vi "Adjacent Locations.vi"(2 "Current Location":cdb) -> (5 "4 Adjacent Locations":T2, 6 "8 Adjacent Locations":T1)   [LabVIEW 2020]
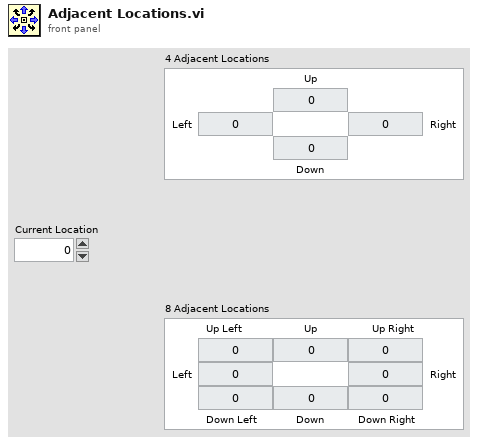
[diagram p1: front panel]
types:
  T1 = cluster{"Up":cdb, "Down":cdb, "Right":cdb, "Left":cdb, "Up Right":cdb, "Up Left":cdb, "Down Right":cdb, "Down Left":cdb}
  T2 = cluster{"Up":cdb, "Down":cdb, "Right":cdb, "Left":cdb}
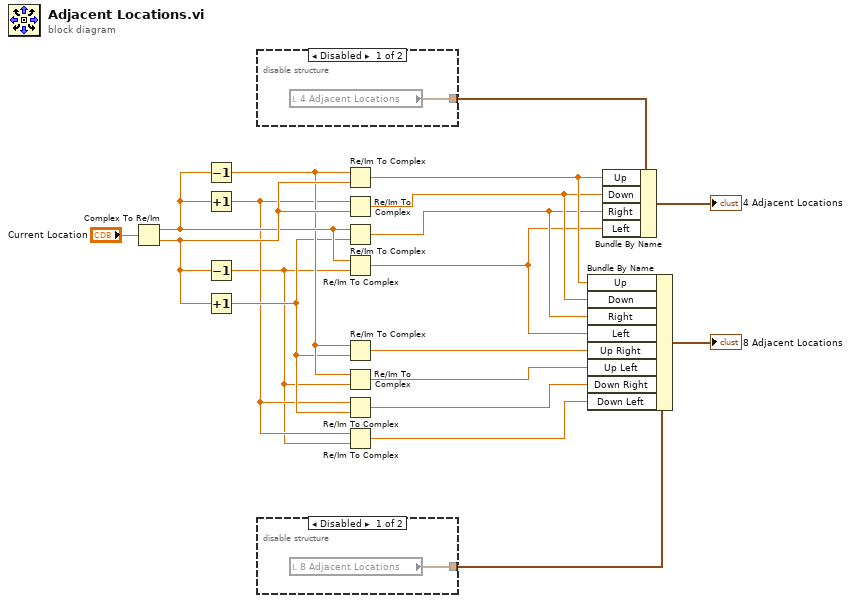
[diagram p0: block diagram]
diagram:
  n1 = Complex To Re/Im(x + iy="Current Location") -> (x=w18:dbl, y=w19:dbl)
  n2 = Decrement(x=w18) -> (x-1=w7:dbl)
  n3 = Increment(x=w18) -> (x+1=w5:dbl)
  n4 = Decrement(x=w19) -> (x-1=w4:dbl)
  n5 = Increment(x=w19) -> (x+1=w6:dbl)
  n6 = disable-structure shown="Disabled" {
    disable-tunnel: [w20 _] -> w15
    frame Disabled {
      n7 = local read "4 Adjacent Locations"() -> (w20:T2)
    }
    frame Enabled {
    }
  }
  n8 = disable-structure shown="Disabled" {
    disable-tunnel: [w21 _] -> w14
    frame Disabled {
      n9 = local read "8 Adjacent Locations"() -> (w21:T1)
    }
    frame Enabled {
    }
  }
  n10 = Re/Im To Complex(1:w19, 2:w7) -> (0:w12:cdb)
  n11 = Re/Im To Complex(1:w19, 2:w5) -> (0:w11:cdb)
  n12 = Re/Im To Complex(1:w6, 2:w18) -> (0:w10:cdb)
  n13 = Re/Im To Complex(1:w4, 2:w18) -> (0:w9:cdb)
  n14 = Re/Im To Complex(1:w6, 2:w7) -> (0:w8:cdb)
  n15 = Re/Im To Complex(1:w4, 2:w7) -> (0:w3:cdb)
  n16 = Re/Im To Complex(1:w6, 2:w5) -> (0:w2:cdb)
  n17 = Re/Im To Complex(1:w4, 2:w5) -> (0:w1:cdb)
  n18 = Bundle By Name(cluster=w14, "Up"=w12, "Down"=w11, "Right"=w10, "Left"=w9, "Up Right"=w8, "Up Left"=w3, "Down Right"=w2, "Down Left"=w1) -> (→"8 Adjacent Locations":T1)
  n19 = Bundle By Name(cluster=w15, "Up"=w12, "Down"=w11, "Right"=w10, "Left"=w9) -> (→"4 Adjacent Locations":T2)
